vi "4431_Voltage_Update.vi"(1 "4431 output":dbl(slide)=-0.0 min=-3.5 max=3.5 scale=-3.5..3.5, 8 "error in":errorcluster, 9 "Amplified output":dbl(slide) min=-50.0 max=50.0 scale=-45.0..45.0, 11 "Physical Channel(s)":tag="Dev2/ao0") -> (0 "error out":errorcluster)   [LabVIEW 2016, in "Transport.lvclass"]
doc: "This example demonstrates how to generate a finite amount of data from a buffer in your computer's memory."
uses:
  Transport.lvclass
  <vilib>/DAQmx/write.llb/DAQmx Write (Analog Wfm 1Chan NSamp).vi
  <vilib>/DAQmx/create/channels.llb/DAQmx Create Channel (AO-Voltage-Basic).vi
  <vilib>/DAQmx/configure/timing.llb/DAQmx Timing (Sample Clock).vi
  <vilib>/DAQmx/miscellaneous.llb/DAQmx Fill In Error Info.vi
  <resource>/objmgr/daqmx.rc
panel:
  in  "Amplifier Gain":dbl=-15.0
  in  "Max Voltage":dbl=3.5
  in  "Min Voltage":dbl=-3.5 min=-3.5 max=0.0
  # "Waveform Settings"
  # "Channel Settings"
  # "Instructions"
  # "-This VI will set a DC output to a NI USB-4431 DSA DAQ\n-The absolute limits are +/- 3.5 V\n- The voltage will be maintained even when the VI is not running & if LabVIEW is shutdown"
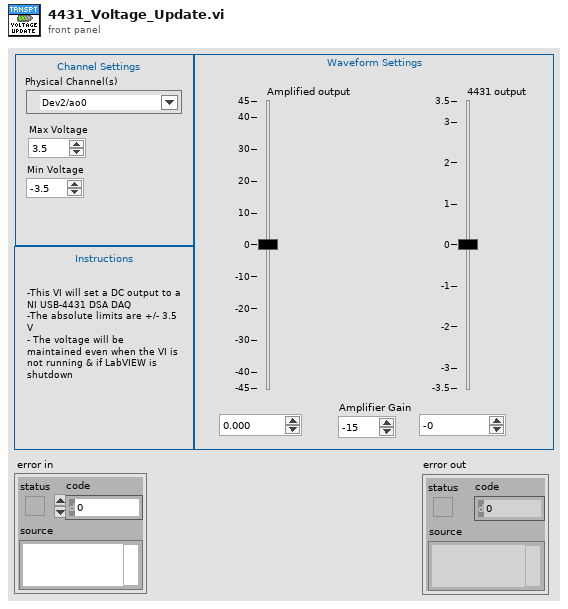
[diagram p1: front panel]
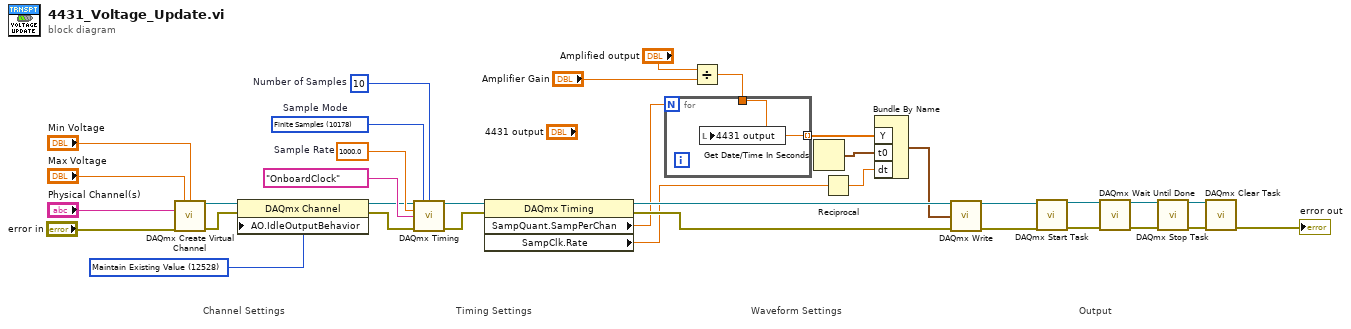
[diagram p0: block diagram]
diagram:
  w22 = 10  # Number of Samples
  w30 = 1000.0  # Sample Rate
  w14 = 12528 items=["Zero Volts"=12526, "High-Impedance"=12527, "Maintain Existing Value"=12528] ("AO.IdleOutputBehavior")
  w34 = 10178 items=["Finite Samples"=10178, "Continuous Samples"=10123, "Hardware Timed Single Point"=12522]  # Sample Mode
  # "Output"
  # "Waveform Settings"
  # "Timing Settings"
  # "Channel Settings"
  n1 = call-poly <vilib>:"DAQmx Create Virtual Channel.vi"("maximum value"="Max Voltage", "minimum value"="Min Voltage", "physical channels"="Physical Channel(s)", "error in"="error in") -> ("task out"=w33:refnum<k21>, "error out"=w16:errorcluster)  [unwired: 10 in]
  n2 = property class="DAQmx Channel"(reference=w33, error in=w16, "AO.IdleOutputBehavior"=w14) -> (reference out=w17:refnum<k21>, error out=w15:errorcluster)
  n3 = call-poly <vilib>:"DAQmx Timing.vi"("task/channels in"=w17, "sample mode"=w34, "samples per channel"=w22, "rate"=w30, "source"=tag "OnboardClock" ("Sample Clock Source"), "error in"=w15) -> ("task out"=w35:refnum<k21>, "error out"=w9:errorcluster)  [unwired: 8 in]
  n4 = property class="DAQmx Timing"(reference=w35, error in=w9) -> (reference out=w27:refnum<k21>, error out=w10:errorcluster, "SampQuant.SampPerChan"=w7:dbl, "SampClk.Rate"=w6:dbl)
  n5 = Divide(x="Amplified output", y="Amplifier Gain") -> (x/y=w3:dbl)
  n6 = for {
    N: w7 -> [_]
    tunnel: [w36] -> w13 mode=indexing
    tunnel: w3 -> [w36]
    n7 = local write "4431 output"(w36) -> ()
  }
  n8 = Get Date/Time In Seconds() -> (seconds since 1Jan1904=w8:timestamp)
  n9 = Reciprocal(x=w6) -> (1/x=w12:dbl)
  n10 = Bundle By Name("Y"=w13, "t0"=w8, "dt"=w12) -> (w11:waveform(dbl))  [unwired: 1 in]
  n11 = call-poly <vilib>:"DAQmx Write.vi"("task/channels in"=w27, "data"=w11, "error in"=w10) -> ("task out"=w26:refnum<k21>, "error out"=w25:errorcluster)  [unwired: 10 in, 1 out]
  n12 = call <vilib>:"DAQmx Start Task.vi"("task/channels in"=w26, "error in"=w25) -> ("task out"=w24:refnum<k21>, "error out"=w23:errorcluster)  [unwired: 12 in]
  n13 = call <vilib>:"DAQmx Wait Until Done.vi"("task/channels in"=w24, "error in"=w23) -> ("task out"=w19:refnum<k21>, "error out"=w18:errorcluster)  [unwired: 12 in]
  n14 = call <vilib>:"DAQmx Stop Task.vi"("task/channels in"=w19, "error in"=w18) -> ("task out"=w21:refnum<k21>, "error out"=w20:errorcluster)  [unwired: 12 in]
  n15 = call <vilib>:"DAQmx Clear Task.vi"("task in"=w21, "error in"=w20) -> ("error out"=→"error out":errorcluster)  [unwired: 13 in]
